vi "prompt.vi"(0 "Enable":bool=TRUE, 5 "error in (no error)":errorcluster) -> (17 "Code":string, 18 "OK":bool, 19 "error out":errorcluster)   [LabVIEW 2019]
doc: "Displays a standard dialog box that prompts users to enter information, such as a user name and password.\n--------------------\n\nThis Express VI is configured as follows:\n\nMessage to Display to the User:Code.py not found. Enter your code here. \nThe inputs are: \nText Entry Box: Code"
panel:
  in  "Code":string
  out "String":string="Code.py not found. Enter your code here. "
  in  "Cancel":bool
  in  "OK2":bool
  in  "OK1":bool
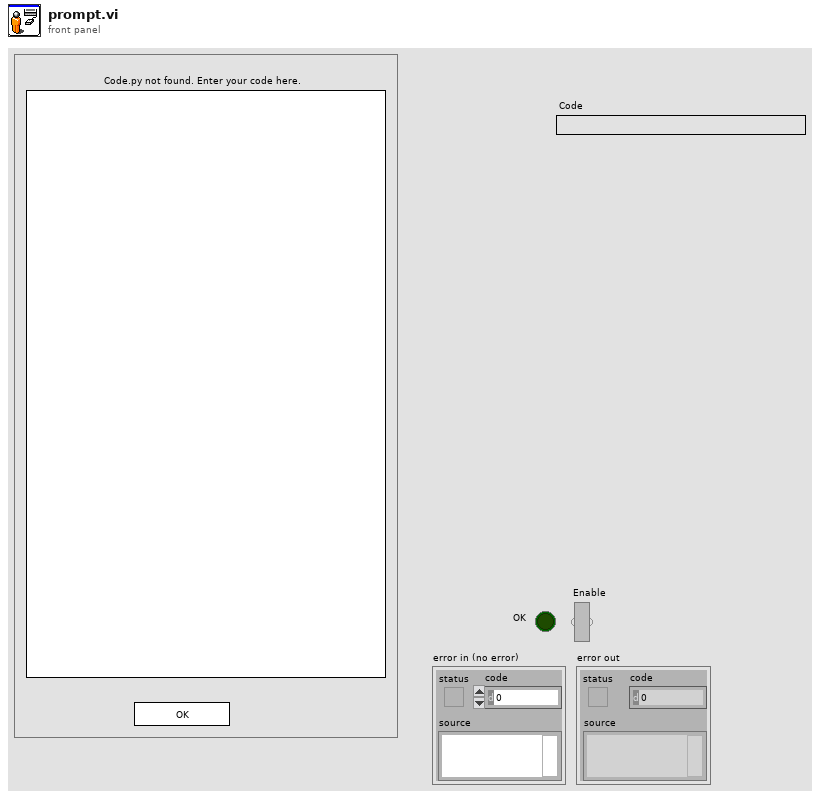
[diagram p1: front panel]
types:
  T1 = cluster{"Input Name":string, "Input Data Type":i32}[]
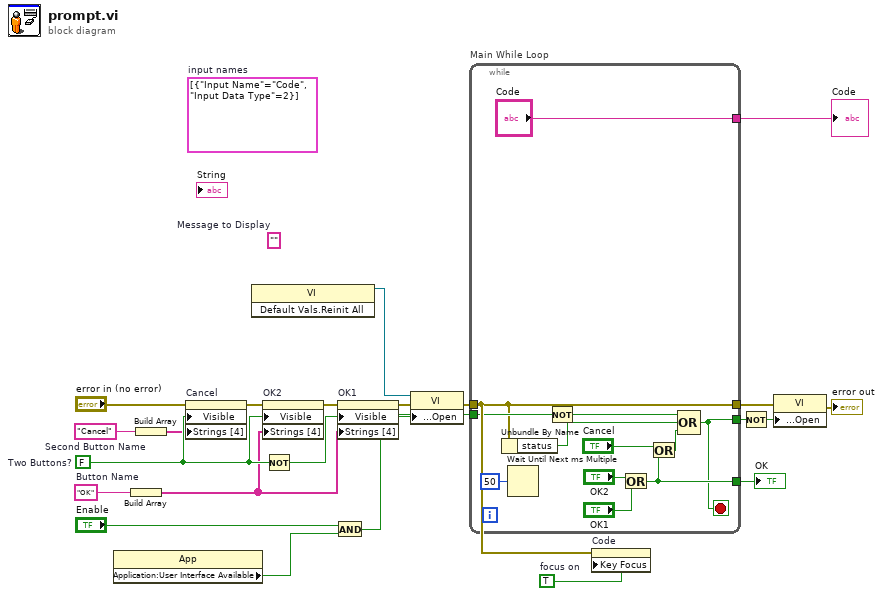
[diagram p0: block diagram]
diagram:
  w1 = TRUE  # focus on
  (unwired) T1 [{"Input Name"="Code", "Input Data Type"=2}]  # input names
  w14 = "Cancel"  # Second Button Name
  w12 = "OK"  # Button Name
  (unwired) ""  # Message to Display
  w22 = FALSE  # Two Buttons?
  n1 = property class="App"() -> ("Application:User Interface Available"=w4:bool)  [unwired: 2 in, 2 out]
  n2 = Build Array(w12) -> (w13:string[])
  n3 = Build Array(w14) -> (w15:string[])
  n4 = property on="Cancel" class="Bool"(error in="error in (no error)", "Visible"=w22, "Strings [4]"=w15) -> (error out=w19:errorcluster)  [unwired: 1 in, 1 out]
  n5 = invoke class="VI" method="Default Vals.Reinit All"() -> (reference out=w3:refnum<vi>)  [unwired: 3 in, 2 out]
  n6 = property on="OK2" class="Bool"(error in=w19, "Visible"=w22, "Strings [4]"=w13) -> (error out=w18:errorcluster)  [unwired: 1 in, 1 out]
  n7 = Not(x=w22) -> (.not. x?=w20:bool)
  n8 = And(x="Enable", y=w4) -> (x .and. y?=w5:bool)
  n9 = property on="OK1" class="Bool"(error in=w18, "Visible"=w20, "Strings [4]"=w13) -> (error out=w11:errorcluster)  [unwired: 1 in, 1 out]
  n10 = property class="VI"(reference=w3, error in=w11, "Front Panel Window:Open"=w5) -> (error out=w10:errorcluster)  [unwired: 1 out]
  n11 = while "Main While Loop" {
    tunnel: [w31] -> w21
    tunnel: w5 -> [w29]
    tunnel: [w27] -> w16
    tunnel: w10 -> [w26]
    tunnel: [w26] -> w8
    tunnel: ["Code"] -> w2
    stop <- w27 stop-if-true
    n12 = Unbundle By Name(w26) -> ("status"=w24:bool)
    n13 = Wait Until Next ms Multiple(millisecond multiple=u32 50) -> ()  [unwired: 1 out]
    n14 = Not(x=w29) -> (.not. x?=w28:bool)
    n15 = Or(x="OK2", y="OK1") -> (x .or. y?=w31:bool)
    n16 = Or(x="Cancel", y=w31) -> (x .or. y?=w25:bool)
    n17 = Compound Arithmetic op=OR(w28, w24, w25) -> (w27:bool)
  }
  "OK" <- w21
  "Code" <- w2
  n18 = property on="Code" class="Str"(error in=w10, "Key Focus"=w1) -> ()  [unwired: 1 in, 2 out]
  n19 = Not(x=w16) -> (.not. x?=w17:bool)
  n20 = property class="VI"(error in=w8, "Front Panel Window:Open"=w17) -> (error out=→"error out":errorcluster)  [unwired: 1 in, 1 out]
